vi "Update Status.vi"(8 "error in (no error)":errorcluster, 11 "Transfer Group in":refnum<class "Transfer Group.lvclass">) -> (0 "error out":errorcluster, 3 "Transfer Group out":refnum<class "Transfer Group.lvclass">)   [LabVIEW 2017, in "DSF Core.lvlib" / "Transfer Group.lvclass"]
uses:
  Transfer Group.lvclass
  Status/Status Data.ctl
  Typedefs/DSF Direction.ctl
  Transfer Group.lvclass/Transfer Group.ctl
  Status/Status Pointer.lvclass
  Performance/Performance.lvclass
  DSF Core.lvlib
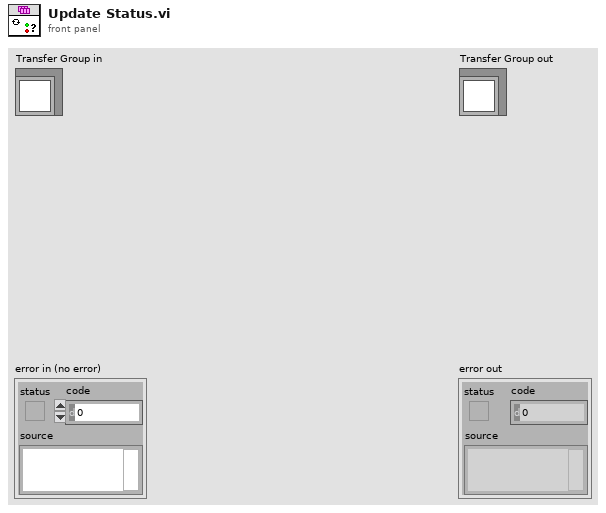
[diagram p1: front panel]
types:
  T1 = typedef "DSF Core.lvlib/DSF Direction.ctl" = enum8{"Tx", "Rx"}
  T2 = typedef "DSF Core.lvlib/Status Pointer.lvclass/Status Data.ctl" = cluster{"iteration":u64, "late count":i32, "duration":u32}
  T3 = typedef "DSF Core.lvlib/Timing Status Pointer.lvclass/Timing Status Data.ctl" = cluster{"rx start time":u32, "rx end time":u32, "tx start time":u32, "tx end time":u32, "cycle start time":u32, "cycle end time":u32, "prev start time":u32}
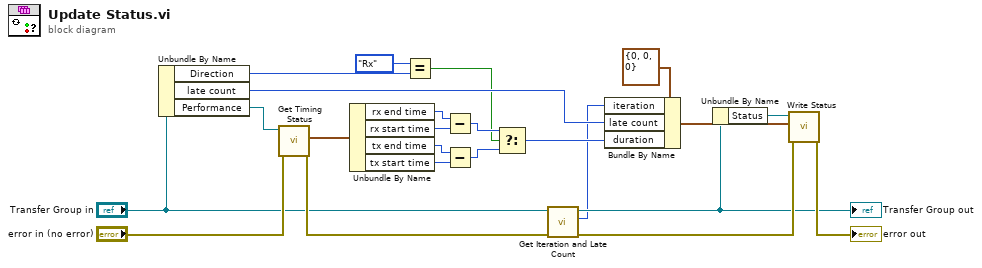
[diagram p0: block diagram]
diagram:
  n1 = Unbundle By Name("Transfer Group in") -> ("Direction"=w9:T1, "late count"=w19:i32, "Performance"=w18:refnum<class "Performance.lvclass">)
  n2 = call "Get Timing Status.vi"("error in (no error)"="error in (no error)", "Framework Performance in"=w18) -> ("error out"=w23:errorcluster, "timing status"=w17:T3)  [unwired: 7 in, 1 out]
  n3 = Unbundle By Name(w17) -> ("rx end time"=w15:u32, "rx start time"=w16:u32, "tx end time"=w14:u32, "tx start time"=w13:u32)
  n4 = Equal?(x=DSF_Direction."Rx", y=w9) -> (x = y?=w7:bool)
  n5 = Subtract(x=w15, y=w16) -> (x-y=w11:u32)
  n6 = Subtract(x=w14, y=w13) -> (x-y=w10:u32)
  n7 = Select(t=w11, s=w7, f=w10) -> (s? t:f=w6:u32)
  n8 = call "Get Iteration and Late Count.vi"("error in (no error)"=w23, "Transfer Group in"="Transfer Group in") -> ("error out"=w20:errorcluster, "iteration"=w1:u64, "Transfer Group out"=w3:refnum<class "Transfer Group.lvclass">)  [unwired: 6 in, 1 out]
  "Transfer Group out" <- w3
  n9 = Bundle By Name(cluster=T2 {"iteration"=0, "late count"=0, "duration"=0} ("status"), "iteration"=w1, "late count"=w19, "duration"=w6) -> (w12:T2)
  n10 = Unbundle By Name(w3) -> ("Status"=w2:refnum<class "Status Pointer.lvclass">)
  n11 = call "Write Status.vi"("error in (no error)"=w20, "status"=w12, "status pointer in"=w2) -> ("error out"=→"error out":errorcluster)  [unwired: 7 in, 1 out]
